vi "Host Image Acquisition Loop.vi"(8 "error in":errorcluster, 11 "Image Reference":refnum<vi>) -> (0 "error out":errorcluster)   [LabVIEW 2013]
doc: "Loop handles the image acquisition communication to FPGA.\nInitialize - Queues up the intialize states\n\nExit"
uses:
  Host Image Acquisition Module Enum.ctl
  Message Passing/MsgQ Loops enum.ctl
  Image Acquisition Settings FG Enum.ctl
  System Status/Status FG Enum.ctl
  Globals/Simulation Settings Global.vi
  Common/State Machines/State Machine Lib.lvlib
  Message Passing/Main MsgQ.lvlib
panel:
  out "State":string
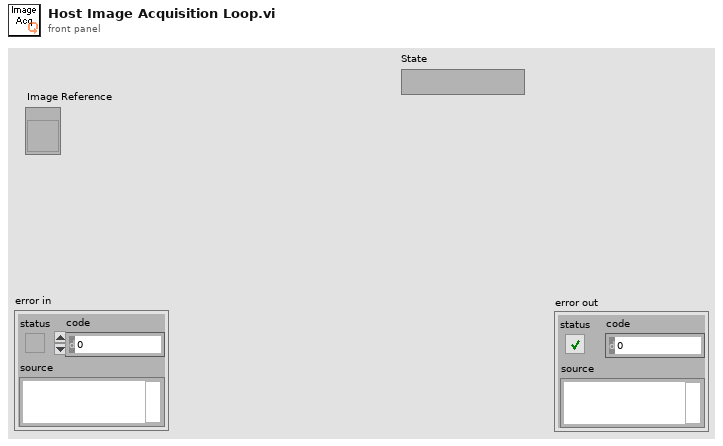
[diagram p1: front panel]
types:
  T1 = typedef "State Machine Lib.lvlib/STATE cluster.ctl" = cluster{"State":string, "Parameters":variant}
  T2 = typedef "Host Image Acquisition Module Enum.ctl" = enum16{"Open FPGA", "Initialize DMA FIFO", "Load Sim Images", "Initialize Acquisition", "Update Sector Parameters", "Start Acquisition", "Aquire Image", "Read Averages", "Cancel Acquisition", "Close FPGA"}
  T3 = typedef "Main MsgQ.lvlib/MsgQ Loops enum.ctl" = enum16{"User Interface", "Image Acq"}
  T4 = typedef "Image Acquisition Settings FG Enum.ctl" = enum16{"Read", "Write"}
  T5 = typedef "Status FG Enum.ctl" = enum16{"Reset", "Read", "Write"}
  T6 = typedef "Simulation Settings Cluster.ctl" = cluster{"Sim Enabled?":bool, "Sim Path":path}
  T7 = typedef "IMAQ Image.ctl" = refnum<image>
  T8 = typedef "Acquisition Settings Cluster.ctl" = cluster{"Image Width":u32, "Image Height":u32, "Frames To Acquire":u32, "Signal Mapping":enum8{"Standard", "Basler 10-tap", "Vosskühler 10-tap"}, "DMA Buffer Size\n(In Images)":u32}
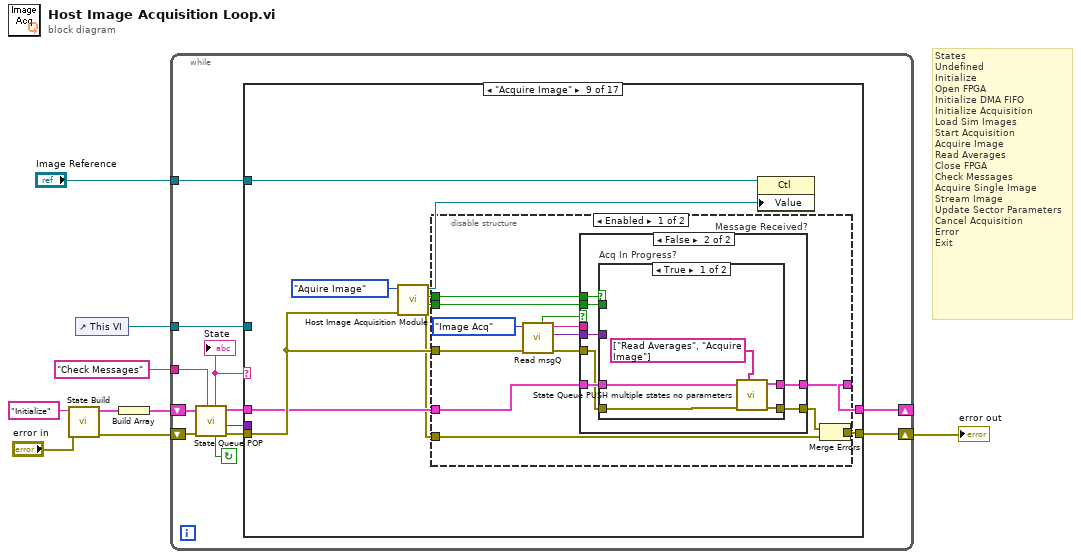
[diagram p0: block diagram]
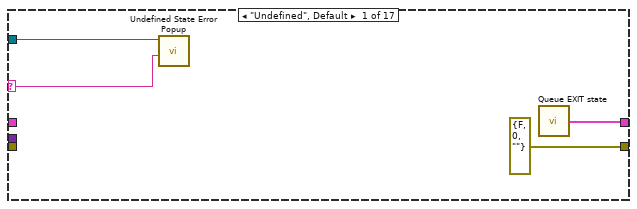
[diagram p2: hidden frame]
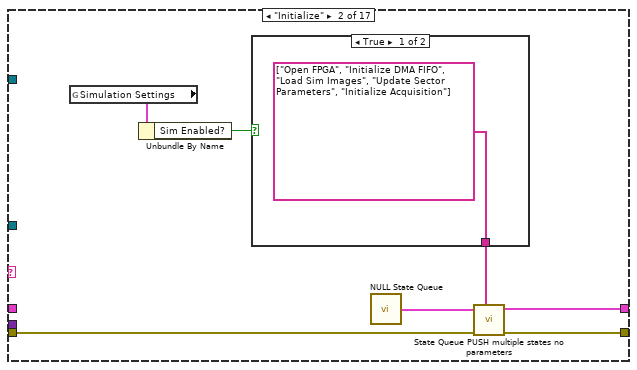
[diagram p3: hidden frame]
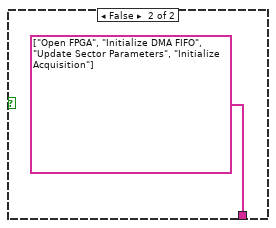
[diagram p4: hidden frame]
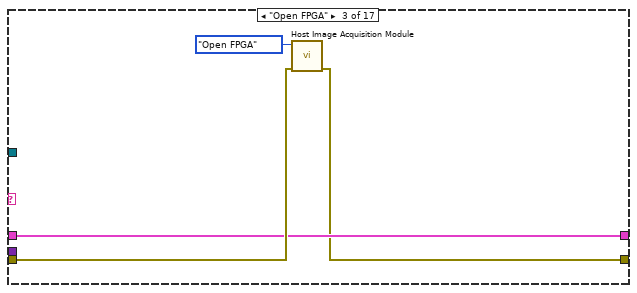
[diagram p5: hidden frame]
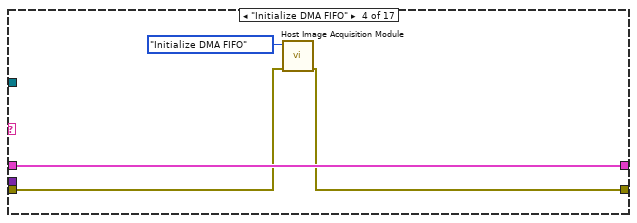
[diagram p6: hidden frame]
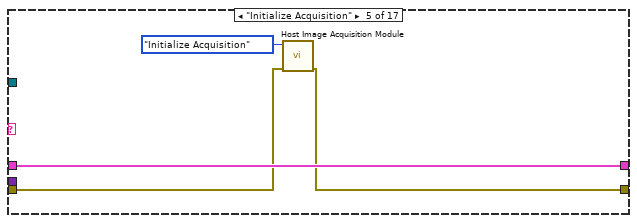
[diagram p7: hidden frame]
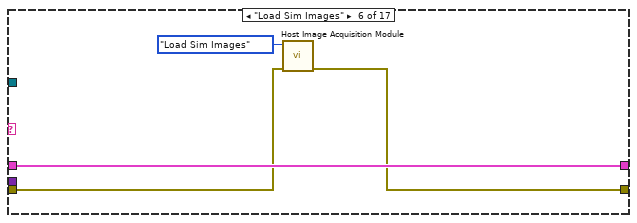
[diagram p8: hidden frame]
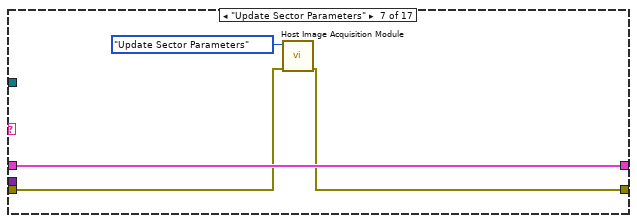
[diagram p9: hidden frame]
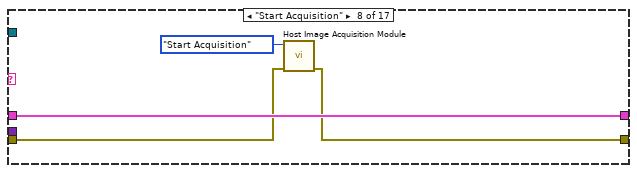
[diagram p10: hidden frame]
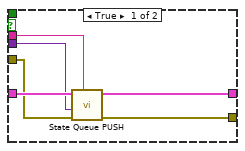
[diagram p11: hidden frame]
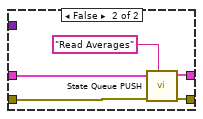
[diagram p12: hidden frame]
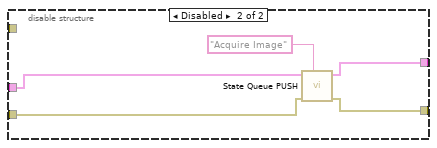
[diagram p13: hidden frame]
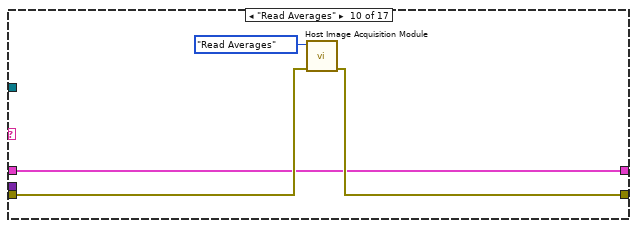
[diagram p14: hidden frame]
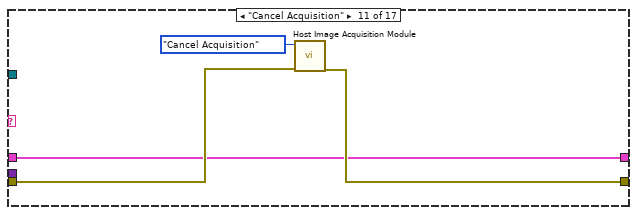
[diagram p15: hidden frame]
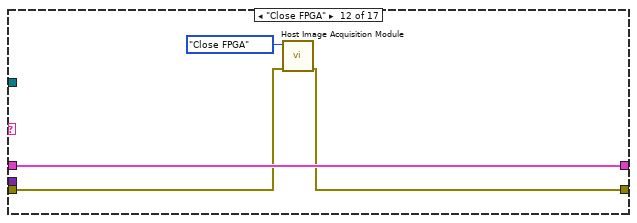
[diagram p16: hidden frame]
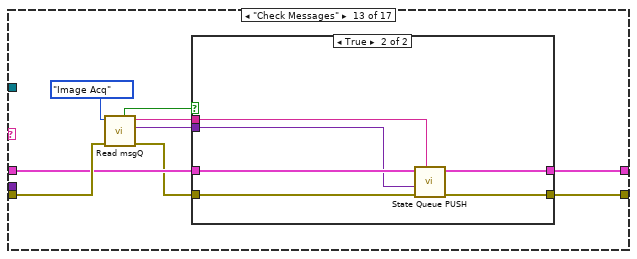
[diagram p17: hidden frame]
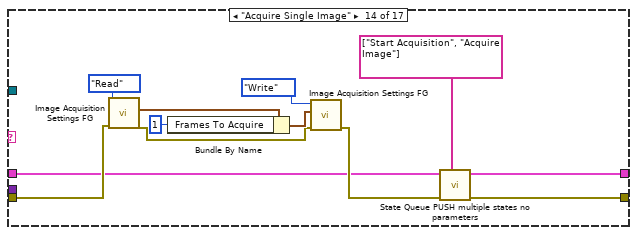
[diagram p19: hidden frame]
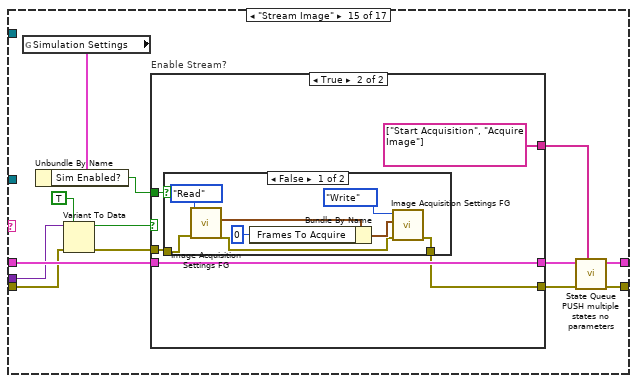
[diagram p20: hidden frame]
diagram:
  # "States\nUndefined\nInitialize\nOpen FPGA\nInitialize DMA FIFO\nInitialize Acquisition\nLoad Sim Images\nStart Acquisition\nAcquire Image\nRead Averages\nClose FPGA\nCheck Messages\nAcquire Single Image\nStream Image\nUpdate Sector Parameters\nCancel Acquisition\nError\nExit"
  n1 = call "State Build.vi"("error in (no error)"="error in", "State"="Initialize") -> ("error out"=w5:errorcluster, "State Out"=w7:T1)  [unwired: 8 in]
  n2 = control-ref of="This VI"() -> (w2:refnum<vi>)
  n3 = Build Array(w7) -> (w6:T1[])
  n4 = while {
    shift-right: [w14] -> _
    shift-left: w6 -> [w21]
    shift-right: [w13] -> w3
    shift-left: w5 -> [w20]
    tunnel: "Check Messages" ("Default state") -> [w18]
    tunnel: w2 -> [w12]
    tunnel: "Image Reference" -> [w11]
    stop <- w19 continue-if-true
    n5 = call "State Queue POP.vi"("Default state"=w18, "error in (no error)"=w20, "State que in"=w21) -> ("error out"=w15:errorcluster, "Parameters"=w10:variant, "State que out"=w16:T1[], "Not Exit?"=w19:bool, "State case out"=w17:string)  [unwired: 4 in]
    "State" <- w17
    n6 = case shown="\"Acquire Image\"" w17 {
      selector: w17 -> [w24 _ _ _ _ _ _ _ _ _ _ _ _ _ _ _ _]
      tunnel: w16 -> [_ _ w36 w42 w46 w50 w54 w58 w66 w110 w114 w121 w128 w142 w163 w183 w190]
      tunnel: w15 -> [_ w32 w37 w41 w45 w49 w53 w57 w67 w112 w116 w120 w130 w149 w153 w186 w189]
      tunnel: [w23 w29 w36 w42 w46 w50 w54 w58 w65 w110 w114 w121 w127 w140 w158 w183 w190] -> w14
      tunnel: [errorcluster {"status"=FALSE, "code"=0, "source"=""} ("error out") w28 w35 w40 w44 w47 w52 w56 w63 w111 w115 w119 w126 w139 w156 w184 w189] -> w13
      tunnel: w12 -> [w25 _ _ _ _ _ _ _ _ _ _ _ _ _ _ _ _]
      tunnel: w11 -> [_ _ _ _ _ _ _ _ w62 _ _ _ _ _ _ _ _]
      tunnel: w10 -> [_ _ _ _ _ _ _ _ _ _ _ _ _ _ w162 _ _]
      frame "Undefined", Default {
        n7 = call "Undefined State Error Popup.vi"("String"=w24, "This VI (Caller if unwired)"=w25) -> ()  [unwired: 10 in]
        n8 = call "Queue EXIT state.vi"() -> ("Exit State Q"=w23:T1[])  [unwired: 1 in]
      }
      frame "Initialize" {
        n9 = global read "Simulation Settings Global.vi" "Simulation Settings"() -> (w27:T6)
        n10 = Unbundle By Name(w27) -> ("Sim Enabled?"=w26:bool)
        n11 = case shown="True" w26 {
          tunnel: [string[] ["Open FPGA", "Initialize DMA FIFO", "Load Sim Images", "Update Sector Parameters", "Initialize Acquisition"] ("States to queue") string[] ["Open FPGA", "Initialize DMA FIFO", "Update Sector Parameters", "Initialize Acquisition"] ("States to queue")] -> w30
          frame True {
          }
          frame False {
          }
        }
        n12 = call "NULL State Queue.vi"() -> ("NULL State Queue"=w31:T1[])
        n13 = call "State Queue PUSH multiple states no parameters.vi"("States to queue"=w30, "error in (no error)"=w32, "State que in"=w31) -> ("error out"=w28:errorcluster, "State que out"=w29:T1[])  [unwired: 7 in]
      }
      frame "Open FPGA" {
        n14 = call "Host Image Acquisition Module.vi"("error in"=w37, "Operation"=Host_Image_Acquisition_Module_Enum."Open FPGA") -> ("error out"=w35:errorcluster)  [unwired: 3 in, 6 out]
      }
      frame "Initialize DMA FIFO" {
        n15 = call "Host Image Acquisition Module.vi"("error in"=w41, "Operation"=Host_Image_Acquisition_Module_Enum."Initialize DMA FIFO") -> ("error out"=w40:errorcluster)  [unwired: 3 in, 6 out]
      }
      frame "Initialize Acquisition" {
        n16 = call "Host Image Acquisition Module.vi"("error in"=w45, "Operation"=Host_Image_Acquisition_Module_Enum."Initialize Acquisition") -> ("error out"=w44:errorcluster)  [unwired: 3 in, 6 out]
      }
      frame "Load Sim Images" {
        n17 = call "Host Image Acquisition Module.vi"("error in"=w49, "Operation"=Host_Image_Acquisition_Module_Enum."Load Sim Images") -> ("error out"=w47:errorcluster)  [unwired: 3 in, 6 out]
      }
      frame "Update Sector Parameters" {
        n18 = call "Host Image Acquisition Module.vi"("error in"=w53, "Operation"=Host_Image_Acquisition_Module_Enum."Update Sector Parameters") -> ("error out"=w52:errorcluster)  [unwired: 3 in, 6 out]
      }
      frame "Start Acquisition" {
        n19 = call "Host Image Acquisition Module.vi"("error in"=w57, "Operation"=Host_Image_Acquisition_Module_Enum."Start Acquisition") -> ("error out"=w56:errorcluster)  [unwired: 3 in, 6 out]
      }
      frame "Acquire Image" {
        n20 = call "Host Image Acquisition Module.vi"("error in"=w67, "Operation"=Host_Image_Acquisition_Module_Enum."Aquire Image") -> ("error out"=w64:errorcluster, "Image Acquired"=w59:bool, "Acq In Progress"=w60:bool, "Image"=w61:T7)  [unwired: 3 in, 3 out]
        n21 = disable-structure shown="Enabled" {
          disable-tunnel: w67 -> [w79 _]
          disable-tunnel: w66 -> [w76 w106]
          disable-tunnel: [w75 w105] -> w65
          disable-tunnel: w64 -> [w73 w107]
          disable-tunnel: [w72 w108] -> w63
          disable-tunnel: w60 -> [w71 _]
          disable-tunnel: w59 -> [w69 _]
          frame Enabled {
            n22 = call "Read msgQ.vi"("error in"=w79, "MsgQ enum"=MsgQ_Loops_enum."Image Acq") -> ("error out"=w77:errorcluster, "Message Received Parameters"=w70:variant, "Message Received String"=w78:string, "Message Recieved?"=w80:bool)  [unwired: 6 in]
            n23 = case "Message Received?" shown="False" w80 {
              tunnel: w78 -> [w86 _]
              tunnel: w77 -> [w85 w93]
              tunnel: w76 -> [w87 w94]
              tunnel: [w84 w92] -> w74
              tunnel: [w83 w91] -> w75
              tunnel: w71 -> [_ w90]
              tunnel: w70 -> [w82 w89]
              tunnel: w69 -> [_ w88]
              frame True {
                n24 = call "State Queue PUSH.vi"("State case"=w86, "error in (no error)"=w85, "Parameters"=w82, "State que in"=w87) -> ("error out"=w84:errorcluster, "State que out"=w83:T1[])  [unwired: 6 in]
              }
              frame False {
                n25 = case "Acq In Progress?" shown="True" w90 {
                  tunnel: w94 -> [w99 w104]
                  tunnel: w93 -> [w96 w101]
                  tunnel: [w97 w102] -> w92
                  tunnel: [w98 w103] -> w91
                  tunnel: w89 -> [_ _]
                  tunnel: w88 -> [_ _]
                  frame True {
                    n26 = call "State Queue PUSH multiple states no parameters.vi"("States to queue"=string[] ["Read Averages", "Acquire Image"], "error in (no error)"=w96, "State que in"=w99) -> ("error out"=w97:errorcluster, "State que out"=w98:T1[])  [unwired: 7 in]
                  }
                  frame False {
                    n27 = call "State Queue PUSH.vi"("State case"="Read Averages", "error in (no error)"=w101, "State que in"=w104) -> ("error out"=w102:errorcluster, "State que out"=w103:T1[])  [unwired: 7 in]
                  }
                }
              }
            }
            n28 = Merge Errors(w74, w73) -> (w72:errorcluster)
          }
          frame Disabled {
            n29 = call "State Queue PUSH.vi"("State case"="Acquire Image", "error in (no error)"=w107, "State que in"=w106) -> ("error out"=w108:errorcluster, "State que out"=w105:T1[])  [unwired: 7 in]
          }
        }
        n30 = property class="Ctl"(reference=w62, "Value"=w61) -> ()  [unwired: 1 in, 2 out]
      }
      frame "Read Averages" {
        n31 = call "Host Image Acquisition Module.vi"("error in"=w112, "Operation"=Host_Image_Acquisition_Module_Enum."Read Averages") -> ("error out"=w111:errorcluster)  [unwired: 3 in, 6 out]
      }
      frame "Cancel Acquisition" {
        n32 = call "Host Image Acquisition Module.vi"("error in"=w116, "Operation"=Host_Image_Acquisition_Module_Enum."Cancel Acquisition") -> ("error out"=w115:errorcluster)  [unwired: 3 in, 6 out]
      }
      frame "Close FPGA" {
        n33 = call "Host Image Acquisition Module.vi"("error in"=w120, "Operation"=Host_Image_Acquisition_Module_Enum."Close FPGA") -> ("error out"=w119:errorcluster)  [unwired: 3 in, 6 out]
      }
      frame "Check Messages" {
        n34 = call "Read msgQ.vi"("error in"=w130, "MsgQ enum"=MsgQ_Loops_enum."Image Acq") -> ("error out"=w125:errorcluster, "Message Received Parameters"=w122:variant, "Message Received String"=w124:string, "Message Recieved?"=w129:bool)  [unwired: 6 in]
        n35 = case shown="True" w129 {
          tunnel: w128 -> [w132 w138]
          tunnel: [w132 w137] -> w127
          tunnel: [w131 w136] -> w126
          tunnel: w125 -> [w131 w135]
          tunnel: w124 -> [_ w133]
          tunnel: w122 -> [_ w134]
          frame False {
          }
          frame True {
            n36 = call "State Queue PUSH.vi"("State case"=w133, "error in (no error)"=w135, "Parameters"=w134, "State que in"=w138) -> ("error out"=w136:errorcluster, "State que out"=w137:T1[])  [unwired: 6 in]
          }
        }
      }
      frame "Acquire Single Image" {
        n37 = call "Image Acquisition Settings FG.vi"("error in (no error)"=w149, "Operation"=Image_Acquisition_Settings_FG_Enum."Read") -> ("error out"=w144:errorcluster, "Acquisition Settings Out"=w148:T8)  [unwired: 8 in]
        n38 = Bundle By Name(cluster=w148, "Frames To Acquire"=u32 1) -> (w146:T8)
        n39 = call "Image Acquisition Settings FG.vi"("error in (no error)"=w144, "Acquisition Settings In"=w146, "Operation"=Image_Acquisition_Settings_FG_Enum."Write") -> ("error out"=w143:errorcluster)  [unwired: 7 in, 1 out]
        n40 = call "State Queue PUSH multiple states no parameters.vi"("States to queue"=string[] ["Start Acquisition", "Acquire Image"], "error in (no error)"=w143, "State que in"=w142) -> ("error out"=w139:errorcluster, "State que out"=w140:T1[])  [unwired: 7 in]
      }
      frame "Stream Image" {
        n41 = global read "Simulation Settings Global.vi" "Simulation Settings"() -> (w154:T6)
        n42 = Unbundle By Name(w154) -> ("Sim Enabled?"=w151:bool)
        n43 = Variant To Data(error in=w153, type=TRUE, Variant=w162) -> (data=w160:bool, error out=w152:errorcluster)
        n44 = case "Enable Stream?" shown="True" w160 {
          tunnel: w152 -> [w164 w171]
          tunnel: w163 -> [w165 w170]
          tunnel: [w165 w170] -> w159
          tunnel: [w164 w169] -> w157
          tunnel: [string[] ["Cancel Acquisition"] ("States to queue") string[] ["Start Acquisition", "Acquire Image"] ("States to queue")] -> w155
          tunnel: w151 -> [_ w167]
          frame False {
          }
          frame True {
            n45 = case shown="False" w167 {
              tunnel: w171 -> [w178 w180]
              tunnel: [w172 w180] -> w169
              frame False {
                n46 = call "Image Acquisition Settings FG.vi"("error in (no error)"=w178, "Operation"=Image_Acquisition_Settings_FG_Enum."Read") -> ("error out"=w173:errorcluster, "Acquisition Settings Out"=w177:T8)  [unwired: 8 in]
                n47 = Bundle By Name(cluster=w177, "Frames To Acquire"=u32 0) -> (w175:T8)
                n48 = call "Image Acquisition Settings FG.vi"("error in (no error)"=w173, "Acquisition Settings In"=w175, "Operation"=Image_Acquisition_Settings_FG_Enum."Write") -> ("error out"=w172:errorcluster)  [unwired: 7 in, 1 out]
              }
              frame True {
              }
            }
          }
        }
        n49 = call "State Queue PUSH multiple states no parameters.vi"("States to queue"=w155, "error in (no error)"=w157, "State que in"=w159) -> ("error out"=w156:errorcluster, "State que out"=w158:T1[])  [unwired: 7 in]
      }
      frame "Error" {
        n50 = Unbundle By Name(w186) -> ("source"=w187:string)
        n51 = Concatenate Strings("Error: " ("string"), w187) -> (w182:string)
        n52 = call "Status FG.vi"("Status In"=w182, "Operation"=Status_FG_Enum."Write") -> ()  [unwired: 8 in, 2 out]
        n53 = call "Broadcast Exit.vi"("error in"=errorcluster {"status"=FALSE, "code"=0, "source"=""}) -> ("error out"=w184:errorcluster)  [unwired: 10 in]
      }
      frame "Exit" {
      }
    }
  }
  "error out" <- w3
